vi "LoadChildClassValues.vi"(8 "error in (no error)":errorcluster caption="entrée d'erreur (pas d'erreur)", 11 "MultiHarp150 en entrée":refnum<class "MultiHarp150.lvclass">) -> (0 "error out":errorcluster caption="sortie d'erreur", 3 "MultiHarp150 en sortie":refnum<class "MultiHarp150.lvclass">)   [LabVIEW 2019, in "MultiHarp150.lvclass"]
uses:
  MultiHarp150.lvclass
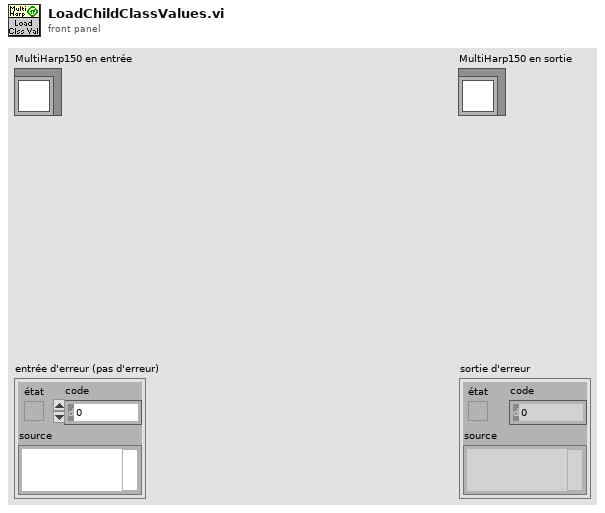
[diagram p1: front panel]
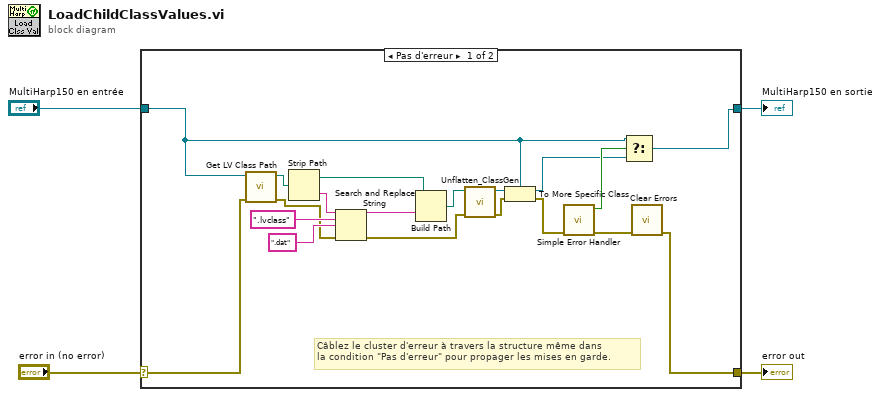
[diagram p0: block diagram]
diagram:
  n1 = case shown="Pas d'erreur" "error in (no error)" {
    selector: "error in (no error)" -> [w6 w25]
    tunnel: [w5 w25] -> w3
    tunnel: [w7 w24] -> w1
    tunnel: "MultiHarp150 en entrée" -> [w8 w24]
    frame No Error {
      # "Câblez le cluster d'erreur à travers la structure même dans\nla condition \"Pas d'erreur\" pour propager les mises en garde."
      n2 = call <vilib>:"Get LV Class Path.vi"("error in (no error)"=w6, "object"=w8) -> ("error out"=w16:errorcluster, "class path"=w21:path)  [unwired: 8 in]
      n3 = Strip Path(path=w21) -> (stripped path=w20:path, name=w19:string)
      n4 = Search and Replace String(input string=w19, search string=".lvclass" ("chaîne recherchée"), replace string=".dat" ("chaîne de remplacement (\"\")"), error in=w16) -> (result string=w15:string, error out=w13:errorcluster)  [unwired: 4 in, 2 out]
      n5 = Build Path(base path=w20, name or relative path=w15) -> (appended path=w14:path)
      n6 = call <userlib>:"Unflatten_ClassGen.vi"("error in (no error)"=w13, "XML File Path"=w14) -> ("sortie d'erreur"=w22:errorcluster, "LabVIEW Object"=w23:refnum<class>)  [unwired: 8 in]
      n7 = To More Specific Class(target class=w8, reference=w23, error in=w22) -> (specific class reference=w9:refnum<class "MultiHarp150.lvclass">, error out=w12:errorcluster)
      n8 = call <vilib>:"Simple Error Handler.vi"("error in (no error)"=w12) -> ("error?"=w10:bool, "error out"=w11:errorcluster)  [unwired: 4 in, 3 out]
      n9 = Select(t=w8, s=w10, f=w9) -> (s? t:f=w7:refnum<class "MultiHarp150.lvclass">)
      n10 = call <vilib>:"Clear Errors.vi"("error in (no error)"=w11) -> ("error out"=w5:errorcluster)  [unwired: 5 in, 1 out]
    }
    frame Error {
    }
  }
  "error out" <- w3
  "MultiHarp150 en sortie" <- w1
